vi "Simulation_Test_NannyTrip(SubVI).vi"(8 "LS_IN":dbl[](array[numeric]), 9 "TC_IN":dbl[](array[numeric]), 10 "PT_IN":dbl[](array[numeric]), 11 "LC_IN":dbl[](array[numeric])) -> (0 "LS_SET_VALUES":dbl[](array[numeric]), 1 "TC_SET_VALUES":dbl[](array[numeric]), 2 "PT_SET_VALUES":dbl[](array[numeric]), 3 "LC_SET_VALUES":dbl[](array[numeric]), 4 "Boolean":bool=TRUE)   [LabVIEW 2020]
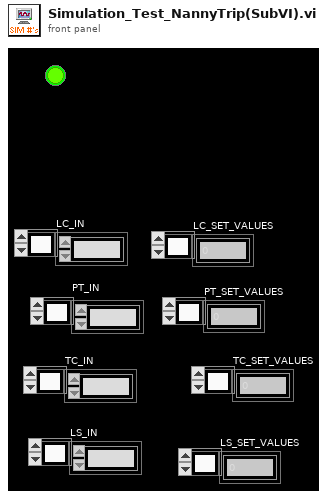
[diagram p1: front panel]
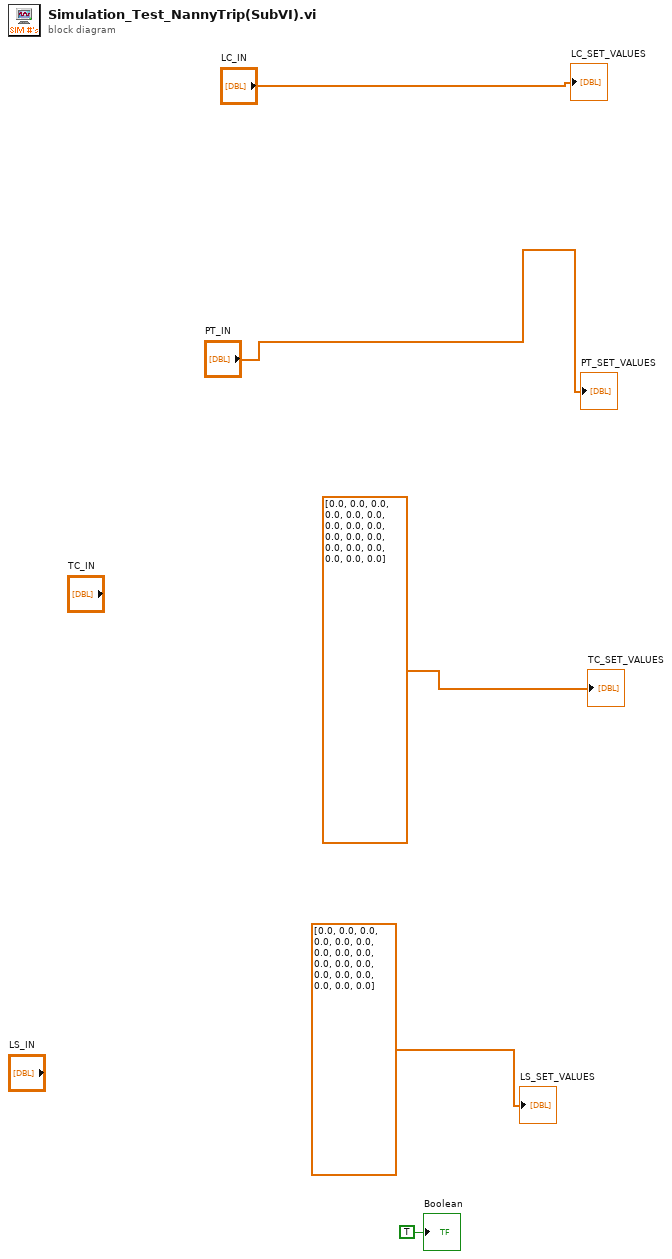
[diagram p0: block diagram]
diagram:
  "TC_SET_VALUES" <- dbl[] [0.0, 0.0, 0.0, 0.0, 0.0, 0.0, 0.0, 0.0, 0.0, 0.0, 0.0, 0.0, 0.0, 0.0, 0.0, 0.0, 0.0, 0.0]
  "PT_SET_VALUES" <- "PT_IN"
  "LC_SET_VALUES" <- "LC_IN"
  "LS_SET_VALUES" <- dbl[] [0.0, 0.0, 0.0, 0.0, 0.0, 0.0, 0.0, 0.0, 0.0, 0.0, 0.0, 0.0, 0.0, 0.0, 0.0, 0.0, 0.0, 0.0]
  "Boolean" <- TRUE
